vi "SetParameter.vi"(8 "error in (no error)":errorcluster, 10 "SetParameter":T1, 11 "ChromaPowerSupply in":refnum<class "ChromaPowerSupply.lvclass">) -> (0 "error out":errorcluster, 2 "StatusUpdates":string[](array[string]), 3 "ChromaPowerSupply out":refnum<class "ChromaPowerSupply.lvclass">)   [LabVIEW 2018, in "AcPwrPlugins.lvlib" / "ChromaPowerSupply.lvclass"]
uses:
  ChromaPowerSupply.lvclass
  AcPwrBaseClass/TypeDefs/SetParameterInputs.ctl
  AcPwrBaseClass/AcPwrBase.lvclass
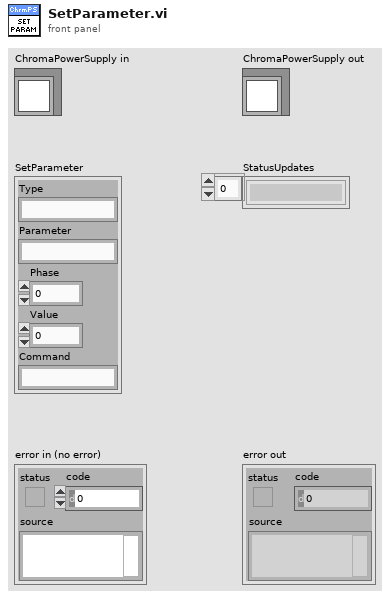
[diagram p1: front panel]
types:
  T1 = typedef "AcPwrPlugins.lvlib/AcPwrBase.lvclass/SetParameterInputs.ctl" = cluster{"Type":string, "Parameter":string, "Phase":i32, "Value":dbl, "Command":string}
  T2 = typedef "AcPwrPlugins.lvlib/ChromaPowerSupply.lvclass/Device(s)Settings.ctl" = cluster{"Phases":cluster{"Handle":string, "Instrument Options":string, "id query (T)":bool, "reset device (T)":bool, "Timing":cluster{"TimingOn":enum16{""}, "Hours":u32, "Minutes":u32, "Seconds":dbl, "CutoffVoltage":dbl}, "Connected":bool, "Output Mode":enum16{"Voltage (DC)", "Current (DC)"}, "Voltage":dbl, "Current":dbl, "Voltage Limit":dbl, "Current Limit":dbl, "Power Protect":dbl, "Current Protect":dbl, "Voltage Protect":dbl}[], "MeasName":string}
  T3 = cluster{"Handle":string, "Instrument Options":string, "id query (T)":bool, "reset device (T)":bool, "Timing":cluster{"TimingOn":enum16{""}, "Hours":u32, "Minutes":u32, "Seconds":dbl, "CutoffVoltage":dbl}, "Connected":bool, "Output Mode":enum16{"Voltage (DC)", "Current (DC)"}, "Voltage":dbl, "Current":dbl, "Voltage Limit":dbl, "Current Limit":dbl, "Power Protect":dbl, "Current Protect":dbl, "Voltage Protect":dbl}[]
  T4 = cluster{"Handle":string, "Instrument Options":string, "id query (T)":bool, "reset device (T)":bool, "Timing":cluster{"TimingOn":enum16{""}, "Hours":u32, "Minutes":u32, "Seconds":dbl, "CutoffVoltage":dbl}, "Connected":bool, "Output Mode":enum16{"Voltage (DC)", "Current (DC)"}, "Voltage":dbl, "Current":dbl, "Voltage Limit":dbl, "Current Limit":dbl, "Power Protect":dbl, "Current Protect":dbl, "Voltage Protect":dbl}
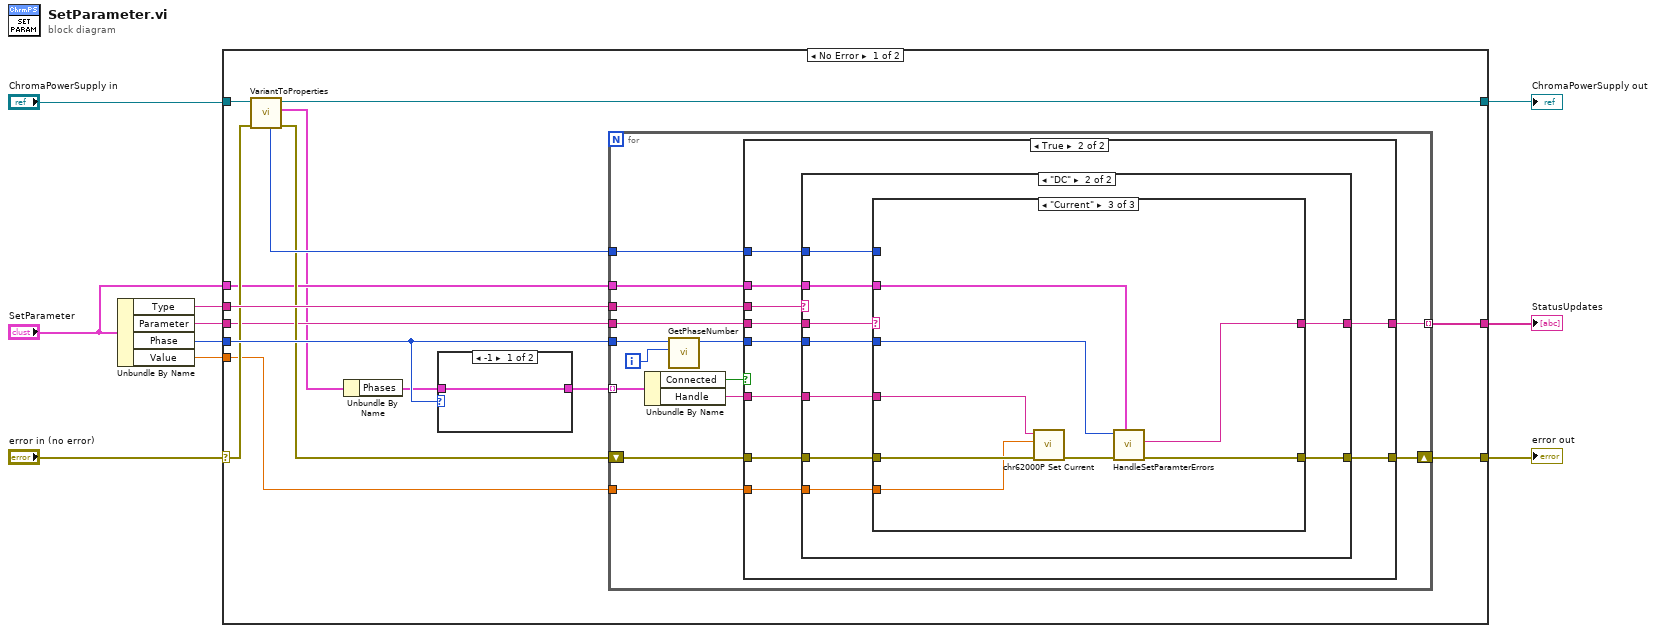
[diagram p0: block diagram]
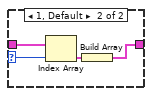
[diagram p2: hidden frame]
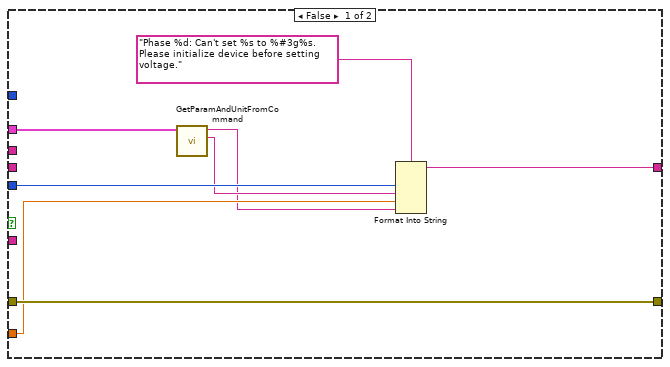
[diagram p3: hidden frame]
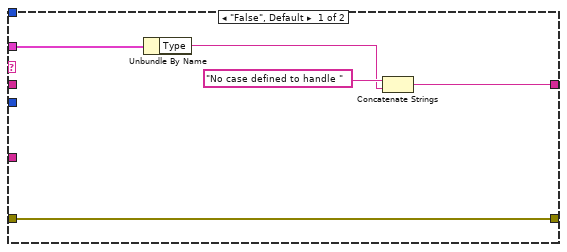
[diagram p4: hidden frame]
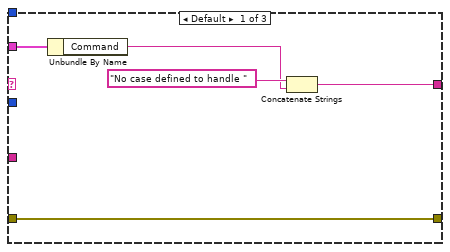
[diagram p5: hidden frame]
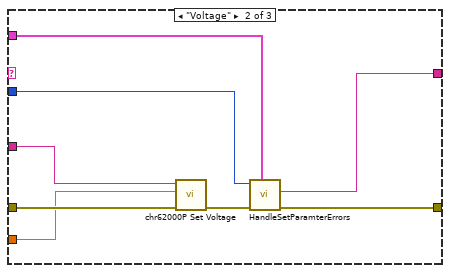
[diagram p6: hidden frame]
diagram:
  n1 = Unbundle By Name("SetParameter") -> ("Type"=w8:string, "Parameter"=w7:string, "Phase"=w10:i32, "Value"=w9:dbl)
  n2 = case shown="No Error" "error in (no error)" {
    selector: "error in (no error)" -> [w18 w99]
    tunnel: "ChromaPowerSupply in" -> [w25 w98]
    tunnel: [w24 w98] -> w5
    tunnel: w10 -> [w21 _]
    tunnel: [w20 _] -> w3
    tunnel: w8 -> [w19 _]
    tunnel: [w16 w99] -> w2
    tunnel: w9 -> [w15 _]
    tunnel: w7 -> [w14 _]
    tunnel: "SetParameter" -> [w13 _]
    frame No Error {
      n3 = call-dynamic "VariantToProperties.vi"("error in (no error)"=w18, "ChromaPowerSupply in"=w25) -> ("error out"=w17:errorcluster, "Device Settings"=w11:T2, "ChromaPowerSupply out"=w24:refnum<class "ChromaPowerSupply.lvclass">, "Measurement Refresh Time (ms)"=w22:u32)  [unwired: 5 in, 1 out]
      n4 = Unbundle By Name(w11) -> ("Phases"=w12:T3)
      n5 = case shown="-1" w21 {
        selector: w21 -> [_ w27]
        tunnel: w12 -> [w26 w30]
        tunnel: [w26 w28] -> w23
        frame -1 {
        }
        frame 1, Default {
          n6 = Index Array(array=w30, index=w27) -> (element=w29:T4)
          n7 = Build Array(w29) -> (w28:T3)
        }
      }
      n8 = for {
        tunnel: w23 -> [w44] mode=indexing
        shift-right: [w42] -> w16
        shift-left: w17 -> [w43]
        tunnel: w15 -> [w39]
        tunnel: w22 -> [w38]
        tunnel: w21 -> [w36]
        tunnel: [w34] -> w20 mode=indexing
        tunnel: w19 -> [w33]
        tunnel: w14 -> [w32]
        tunnel: w13 -> [w31]
        i -> [w37]
        n9 = Unbundle By Name(w44) -> ("Connected"=w41:bool, "Handle"=w40:string)
        n10 = call "GetPhaseNumber.vi"("Loop Counter"=w37, "Phase(-1, all) in"=w36) -> ("Phase(-1, all) out"=w35:i32)  [unwired: 9 in]
        n11 = case shown="True" w41 {
          tunnel: w43 -> [w52 w62]
          tunnel: [w52 w61] -> w42
          tunnel: w40 -> [_ w60]
          tunnel: w39 -> [w46 w59]
          tunnel: w38 -> [_ w58]
          tunnel: w35 -> [w51 w57]
          tunnel: [w49 w56] -> w34
          tunnel: w33 -> [_ w55]
          tunnel: w32 -> [_ w54]
          tunnel: w31 -> [w48 w53]
          frame False {
            n12 = call "GetParamAndUnitFromCommand.vi"("SetParameter"=w48) -> ("Parameter"=w47:string, "Unit Label"=w45:string)  [unwired: 9 in]
            n13 = Format Into String(format string="Phase %d: Can't set %s to %#3g%s. Please initialize device before setting voltage.", w51, w47, w46, w45) -> (resulting string=w49:string)  [unwired: 2 in, 1 out]
          }
          frame True {
            n14 = case shown="\"DC\"" w55 {
              tunnel: w62 -> [w63 w76]
              tunnel: [w63 w75] -> w61
              tunnel: w60 -> [_ w74]
              tunnel: w59 -> [_ w73]
              tunnel: w58 -> [_ w72]
              tunnel: w57 -> [_ w71]
              tunnel: [w64 w70] -> w56
              tunnel: w54 -> [_ w69]
              tunnel: w53 -> [w65 w68]
              frame "False", Default {
                n15 = Unbundle By Name(w65) -> ("Type"=w66:string)
                n16 = Concatenate Strings("No case defined to handle " ("string"), w66) -> (w64:string)
              }
              frame "DC" {
                n17 = case shown="\"Current\"" w69 {
                  tunnel: w76 -> [w81 w85 w93]
                  tunnel: [w81 w89 w97] -> w75
                  tunnel: w74 -> [_ w83 w91]
                  tunnel: w73 -> [_ w82 w90]
                  tunnel: w72 -> [_ _ _]
                  tunnel: w71 -> [_ w88 w96]
                  tunnel: [w80 w87 w95] -> w70
                  tunnel: w68 -> [w78 w86 w94]
                  frame Default {
                    n18 = Unbundle By Name(w78) -> ("Command"=w77:string)
                    n19 = Concatenate Strings("No case defined to handle " ("string"), w77) -> (w80:string)
                  }
                  frame "Voltage" {
                    n20 = call <instrlib>:"chr62000P Set Voltage.vi"("error in (no error)"=w85, "Voltage (0.00)"=w82, "instrument handle"=w83) -> ("error out"=w84:errorcluster)  [unwired: 7 in, 1 out]
                    n21 = call "HandleSetParamterErrors.vi"("SetParameter"=w86, "error in (no error)"=w84, "Phase"=w88) -> ("error IO"=w89:errorcluster, "Status Update"=w87:string)  [unwired: 7 in]
                  }
                  frame "Current" {
                    n22 = call <instrlib>:"chr62000P Set Current.vi"("error in (no error)"=w93, "Current (0.00)"=w90, "instrument handle"=w91) -> ("error out"=w92:errorcluster)  [unwired: 7 in, 1 out]
                    n23 = call "HandleSetParamterErrors.vi"("SetParameter"=w94, "error in (no error)"=w92, "Phase"=w96) -> ("error IO"=w97:errorcluster, "Status Update"=w95:string)  [unwired: 7 in]
                  }
                }
              }
            }
          }
        }
      }
    }
    frame Error {
    }
  }
  "error out" <- w2
  "ChromaPowerSupply out" <- w5
  "StatusUpdates" <- w3
